vi "Path FGV.vi"(8 "error in (no error)":errorcluster, 9 "Set?":bool, 10 "Library Path":path) -> (0 "error out (no error)":errorcluster, 2 "Library Path":path)   [LabVIEW 2020, in "lvzstd.lvlib"]
uses:
  lvzstd.lvlib
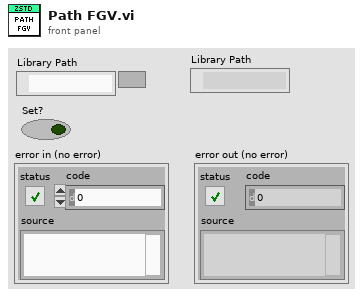
[diagram p1: front panel]
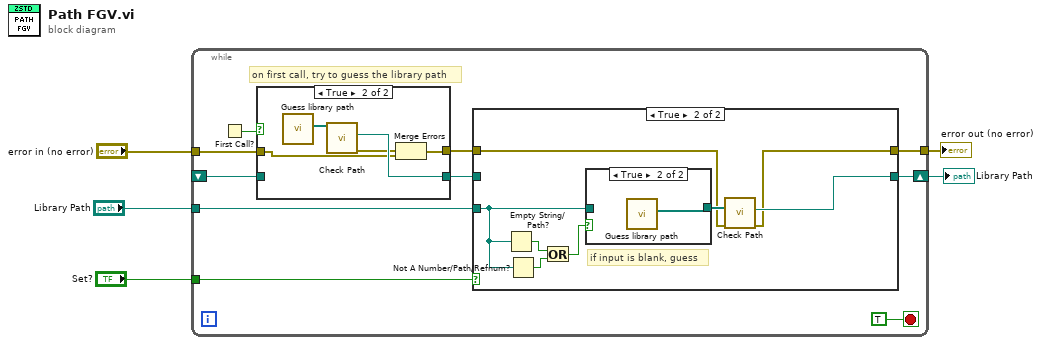
[diagram p0: block diagram]
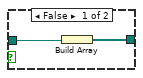
[diagram p4: hidden frame]
diagram:
  n1 = while {
    shift-right: [w12] -> w3
    shift-left: _ -> [w11]
    tunnel: "Set?" -> [w14]
    tunnel: "Library Path" -> [w13]
    tunnel: [w8] -> w1
    tunnel: "error in (no error)" -> [w7]
    stop <- TRUE stop-if-true
    # "on first call, try to guess the library path"
    n2 = First Call?() -> (First Call?: T/F=w6:bool)
    n3 = case shown="True" w6 {
      tunnel: w11 -> [w17 _]
      tunnel: [w17 w22] -> w10
      tunnel: [w16 w18] -> w9
      tunnel: w7 -> [w16 w19]
      frame False {
      }
      frame True {
        n4 = call "Guess library path.vi"() -> ("paths"=w21:path[])  [unwired: 11 in]
        n5 = call "Check Path.vi"("appended array"=w21) -> ("error in (no error)"=w20:errorcluster, "Library Path"=w22:path)  [unwired: 9 in]
        n6 = Merge Errors(w20, w19) -> (w18:errorcluster)
      }
    }
    n7 = case shown="True" w14 {
      tunnel: w13 -> [_ w26]
      tunnel: [w24 w31] -> w12
      tunnel: w10 -> [w24 _]
      tunnel: w9 -> [w23 w30]
      tunnel: [w23 w29] -> w8
      frame False {
      }
      frame True {
        # "if input is blank, guess"
        n8 = Empty String/Path?(string/path=w26) -> (empty?=w27:bool)
        n9 = Not A Number/Path/Refnum?(number/path/refnum=w26) -> (NaN/Path/Refnum?=w28:bool)
        n10 = Or(x=w27, y=w28) -> (x .or. y?=w25:bool)
        n11 = case shown="True" w25 {
          tunnel: w26 -> [w34 _]
          tunnel: [w33 w35] -> w32
          frame False {
            n12 = Build Array(w34) -> (w33:path[])
          }
          frame True {
            n13 = call "Guess library path.vi"() -> ("paths"=w35:path[])  [unwired: 11 in]
          }
        }
        n14 = call "Check Path.vi"("error in (no error)"=w30, "appended array"=w32) -> ("error in (no error)"=w29:errorcluster, "Library Path"=w31:path)  [unwired: 8 in]
      }
    }
  }
  "Library Path" <- w3
  "error out (no error)" <- w1
